vi "Работа с TXT файлом knob вариант 2.vi"() -> ()   [LabVIEW 2021]
panel:
  out "text":string
  in  "Knob":dbl(knob) scale=0.0..10.0
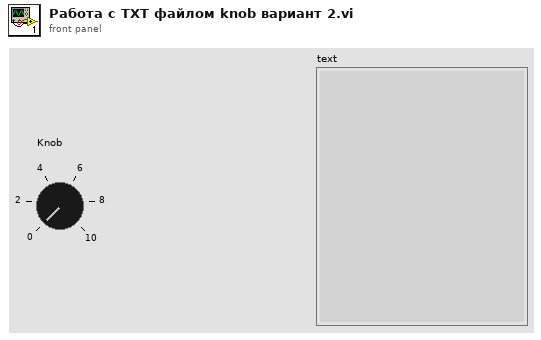
[diagram p1: front panel]
types:
  T1 = enum16{"open", "replace", "create", "open or create", "replace or create", "replace or create with confirmation"}
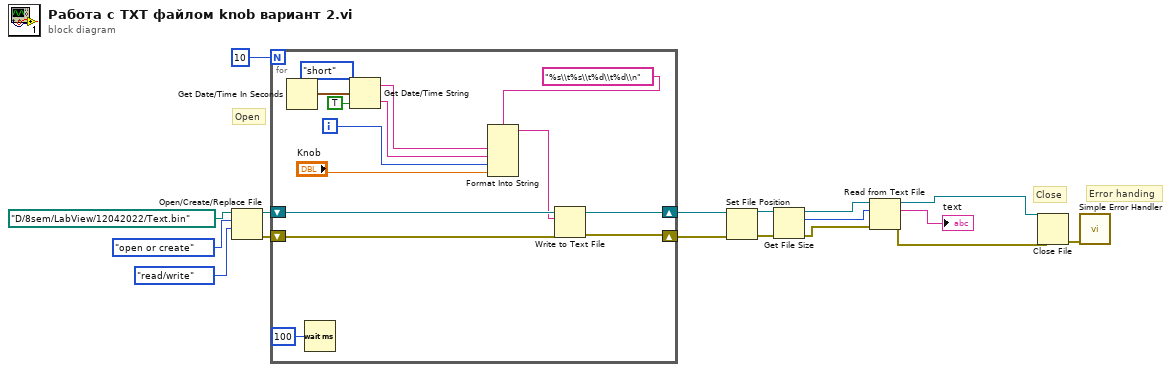
[diagram p0: block diagram]
diagram:
  # "Error handing"
  # "Close"
  # "Open"
  n1 = Open/Create/Replace File(file path (use dialog)=path "D:/8sem/LabView/12042022/Text.bin", operation (0:open)=T1."open or create", access (0:read/write)=enum16{"read/write", "read-only", "write-only"}."read/write") -> (refnum out=w13:refnum<file>, error out=w14:errorcluster)  [unwired: 3 in, 1 out]
  n2 = for {
    N: 10 -> [_]
    shift-right: [w29] -> w10
    shift-left: w14 -> [w27]
    shift-right: [w30] -> w11
    shift-left: w13 -> [w28]
    i -> [w19]
    n3 = Get Date/Time In Seconds() -> (seconds since 1Jan1904=w26:timestamp)
    n4 = Wait (ms)(milliseconds to wait=u32 100) -> ()  [unwired: 1 out]
    n5 = Get Date/Time String(date format (0)=enum16{"short", "long", "abbreviated"}."short", seconds (now)=w26, want seconds? (F)=TRUE) -> (date string=w22:string, time string=w20:string)
    n6 = Format Into String(format string="%s\\t%s\\t%d\\t%d\\n", w22, w20, w19, "Knob") -> (resulting string=w21:string)  [unwired: 2 in, 1 out]
    n7 = Write to Text File(file (use dialog)=w28, text=w21, error in=w27) -> (refnum out=w30:refnum<file>, error out=w29:errorcluster)  [unwired: 1 in, 1 out]
  }
  n8 = Set File Position(refnum=w11, error in=w10) -> (refnum out=w2:refnum<file>, error out=w3:errorcluster)  [unwired: 2 in]
  n9 = Get File Size(file=w2, error in=w3) -> (refnum out=w1:refnum<file>, size (in bytes)=w4:i64, 0:w5:errorcluster)
  n10 = Read from Text File(file (use dialog)=w1, count=w4, error in=w5) -> (refnum out=w8:refnum<file>, text=→"text":string, error out=w9:errorcluster)  [unwired: 1 in, 1 out]
  n11 = Close File(refnum=w8, error in=w9) -> (error out=w15:errorcluster)  [unwired: 1 out]
  n12 = call <vilib>:"Simple Error Handler.vi"("error in (no error)"=w15) -> ()  [unwired: 4 in, 5 out]
